vi "JSON Delta Solenoid Update.vi"(9 "Delta JSON":string, 11 "input":T1={"type"="Solenoid", "device"="", "name"="", "data"={"<output"=FALSE}}) -> (0 "error out":errorcluster, 3 "output":T1={"type"="Solenoid", "device"="", "name"="", "data"={"<output"=FALSE}})   [LabVIEW 2019]
uses:
  Solenoid proto.ctl
  Solenoid Data proto.ctl
panel:
  out "JSON of original":string
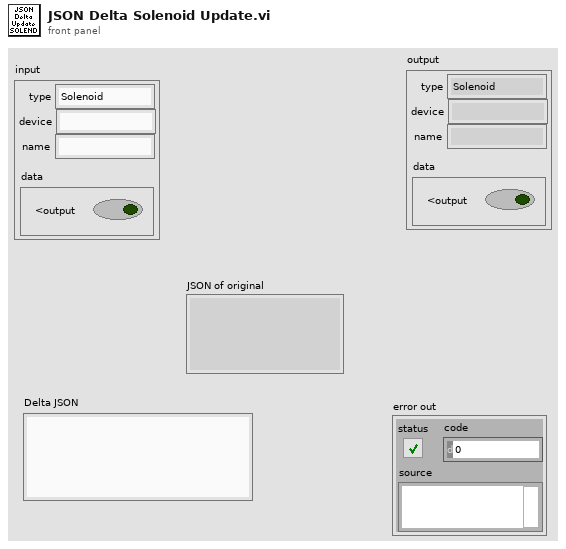
[diagram p1: front panel]
types:
  T1 = typedef "Solenoid proto.ctl" = cluster{"type":string, "device":string, "name":string, "data":T2}
  T2 = typedef "Solenoid Data proto.ctl" = cluster{"<output":bool}
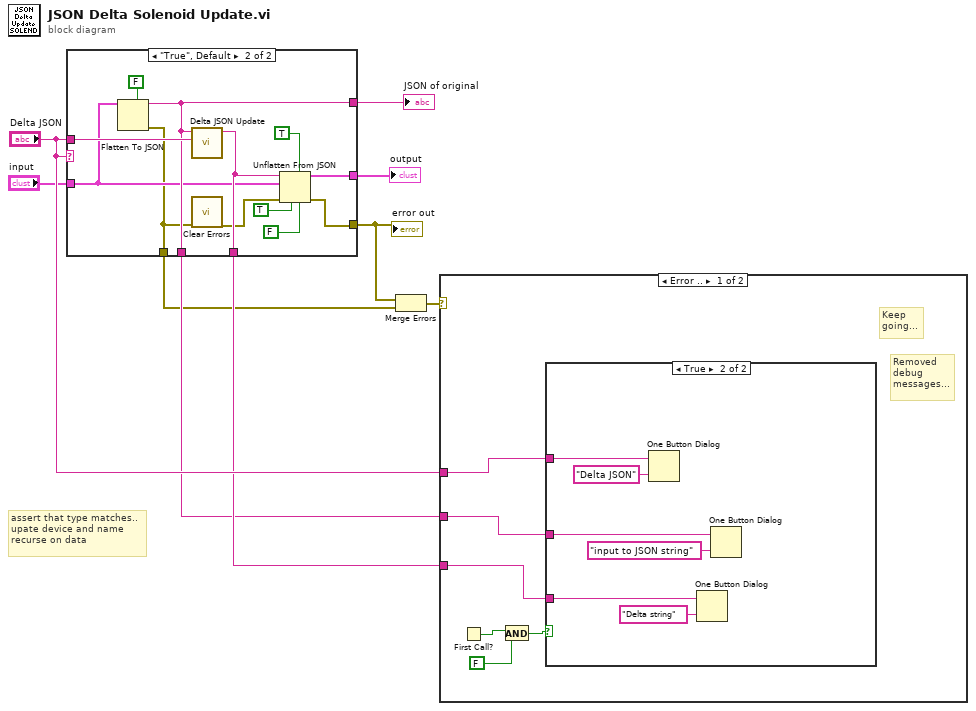
[diagram p0: block diagram]
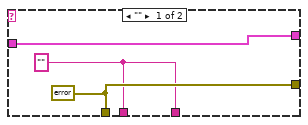
[diagram p4: hidden frame]
diagram:
  # "assert that type matches..\nupate device and name\nrecurse on data"
  n1 = case shown="\"True\", Default" "Delta JSON" {
    tunnel: [_ w18] -> w9
    tunnel: "Delta JSON" -> [_ w23]
    tunnel: [w11 w22] -> w2
    tunnel: "input" -> [w12 w17]
    tunnel: [w12 w20] -> w8
    tunnel: [w10 w19] -> w6
    tunnel: [w10 w18] -> w5
    tunnel: [w11 w14] -> w1
    frame "" {
      w11 = errorcluster {"status"=FALSE, "code"=0, "source"=""} ("error out")
      w10 = "" ("JSON string out")
    }
    frame "True", Default {
      n2 = Flatten To JSON(enable LabVIEW extensions? (T)=FALSE, anything=w17) -> (JSON string=w18:string, 11:w14:errorcluster)  [unwired: 1 in]
      n3 = call "Delta JSON Update.vi"("Delta JSON"=w23, "JSON string in"=w18) -> ("JSON string out"=w19:string)  [unwired: 9 in]
      n4 = call <vilib>:"Clear Errors.vi"("error in (no error)"=w14) -> ("error out"=w13:errorcluster)  [unwired: 5 in, 1 out]
      n5 = Unflatten From JSON(enable LabVIEW extensions? (T)=TRUE, JSON string=w19, type and defaults=w17, default null elements? (F)=TRUE, strict validation? (F)=FALSE, error in (no error)=w13) -> (value=w20:T1, error out=w22:errorcluster)  [unwired: 1 in]
    }
  }
  "JSON of original" <- w9
  "error out" <- w2
  "output" <- w8
  n6 = Merge Errors(w2, w1) -> (w3:errorcluster)
  n7 = case shown="Error .." w3 {
    tunnel: "Delta JSON" -> [w30 _]
    tunnel: w6 -> [w28 _]
    tunnel: w5 -> [w29 _]
    frame Error {
      # "Removed\ndebug\nmessages..."
      # "Keep\ngoing..."
      n8 = First Call?() -> (First Call?: T/F=w27:bool)
      n9 = And(x=w27, y=FALSE) -> (x .and. y?=w25:bool)
      n10 = case shown="True" w25 {
        tunnel: w30 -> [_ w36]
        tunnel: w29 -> [_ w33]
        tunnel: w28 -> [_ w31]
        frame False {
        }
        frame True {
          n11 = One Button Dialog(message=w36, button name ("OK")="Delta JSON") -> ()  [unwired: 1 out]
          n12 = One Button Dialog(message=w31, button name ("OK")="Delta string") -> ()  [unwired: 1 out]
          n13 = One Button Dialog(message=w33, button name ("OK")="input to JSON string") -> ()  [unwired: 1 out]
        }
      }
    }
    frame No Error {
    }
  }
